vi "pH to % v1_0.vi"(1 "Minimum pH":dbl format="%.2f", 2 "Input pH":dbl format="%.2f", 3 "Maximum pH":dbl=14.0 format="%.2f") -> (0 "Output Percentage":dbl format="%.2f")   [LabVIEW 2012]
panel:
  # "pH to %"
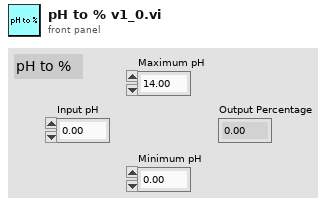
[diagram p1: front panel]
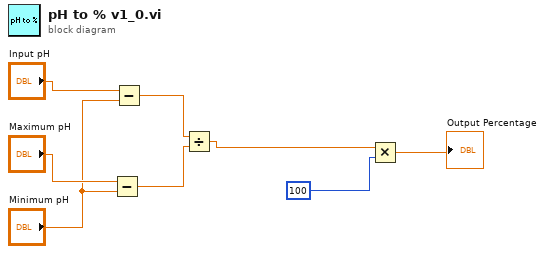
[diagram p0: block diagram]
diagram:
  n1 = Subtract(x="Maximum pH", y="Minimum pH") -> (x-y=w4:dbl)
  n2 = Subtract(x="Input pH", y="Minimum pH") -> (x-y=w5:dbl)
  n3 = Divide(x=w5, y=w4) -> (x/y=w3:dbl)
  n4 = Multiply(x=w3, y=100) -> (x*y=→"Output Percentage":dbl)
